vi "dfd_Check Delay Change.vi"(7 "init in":bool, 8 "error in (no error)":errorcluster, 11 "delay in":i32) -> (0 "error out":errorcluster, 3 "delay out":i32, 5 "init out":bool)   [LabVIEW 2017, in "NI_DigFilter_Process.lvlib"]
uses:
  <vilib>/addons/Digital Filter Design/NI_DigFilter_Process.lvlib
  <vilib>/addons/Digital Filter Design/_Misc.llb/dfd_Error Handlers (Single).vi
  <vilib>/addons/Digital Filter Design/NI_DigFilterLicensed.lvlib
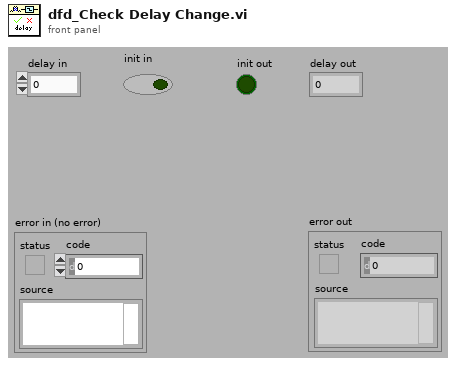
[diagram p1: front panel]
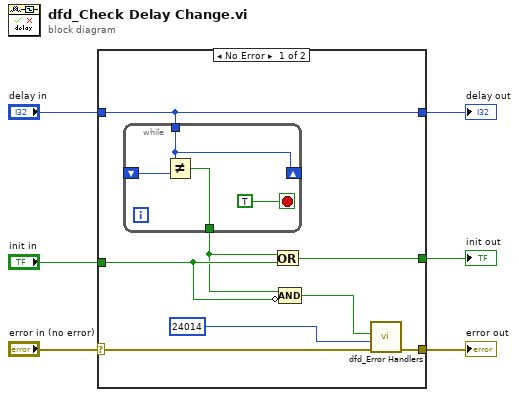
[diagram p0: block diagram]
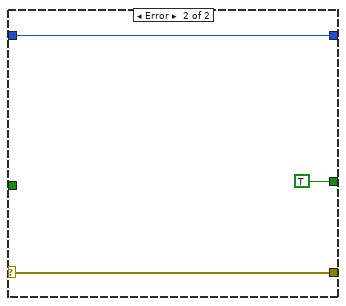
[diagram p2: hidden frame]
diagram:
  n1 = case shown="No Error" "error in (no error)" {
    selector: "error in (no error)" -> [w9 w19]
    tunnel: "init in" -> [w13 _]
    tunnel: [w14 TRUE] -> w2
    tunnel: "delay in" -> [w8 w21]
    tunnel: [w8 w21] -> w6
    tunnel: [w7 w19] -> w1
    frame No Error {
      n2 = while {
        shift-right: [w17] -> _
        shift-left: _ -> [w18]
        tunnel: w8 -> [w17]
        tunnel: [w16] -> w12
        stop <- TRUE stop-if-true
        n3 = Not Equal?(x=w17, y=w18) -> (x != y?=w16:bool)
      }
      n4 = Or(x=w12, y=w13) -> (x .or. y?=w14:bool)
      n5 = Compound Arithmetic op=AND(w12, invert w13) -> (w11:bool)
      n6 = call-poly <vilib>:"dfd_Error Handlers.vi"("error in (no error)"=w9, "error code"=24014 ("WRN_DELAY_INCONSISTENT"), "condition failed?"=w11) -> ("error out"=w7:errorcluster)  [unwired: 8 out]
    }
    frame Error {
    }
  }
  "error out" <- w1
  "init out" <- w2
  "delay out" <- w6
